vi "Level_DSP.vi"(8 "error in (no error)":errorcluster caption="에러 입력(에러 없음)", 9 "Curr":dbl, 10 "Volt":dbl, 11 "VISA resource name":refnum<visa-resource-name>) -> (0 "error out":errorcluster caption="에러 출력", 3 "VISA resource name Out":refnum<visa-resource-name>)   [LabVIEW 2019]
uses:
  f78cf197-b02f-4b1b-bb70-fad094e02e99.vi
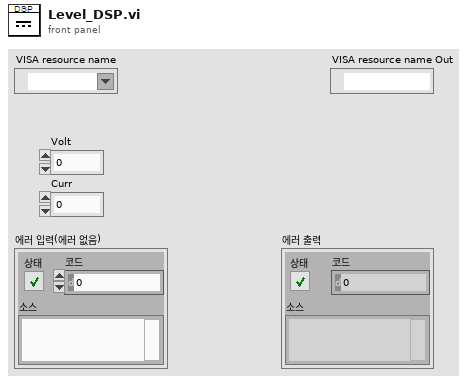
[diagram p1: front panel]
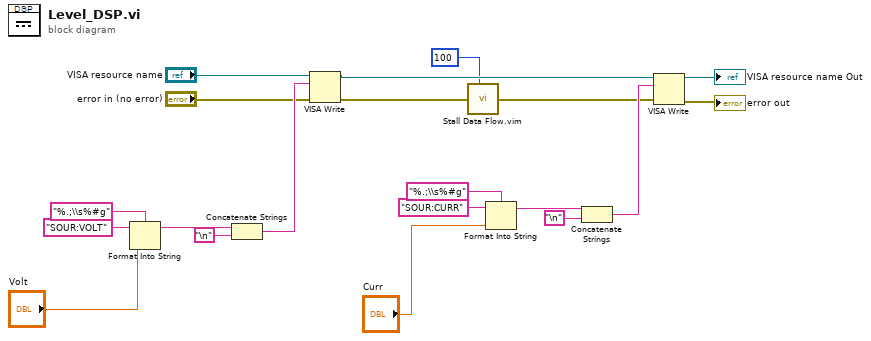
[diagram p0: block diagram]
diagram:
  n1 = Format Into String(format string="%.;\\s%#g", initial string="SOUR:VOLT", "Volt") -> (resulting string=w14:string)  [unwired: 1 in, 1 out]
  n2 = Concatenate Strings(w14, "\n") -> (w19:string)
  n3 = VISA Write(VISA resource name="VISA resource name", write buffer=w19, error in (no error)="error in (no error)") -> (VISA resource name out=w8:refnum<visa-resource-name>, error out=w7:errorcluster)  [unwired: 1 out]
  n4 = call "Stall Data Flow.vim"("value in"=w7, "milliseconds to wait"=u32 100) -> ("value out"=w2:errorcluster)  [unwired: 1 out]
  n5 = Format Into String(format string="%.;\\s%#g", initial string="SOUR:CURR", "Curr") -> (resulting string=w5:string)  [unwired: 1 in, 1 out]
  n6 = Concatenate Strings(w5, "\n") -> (w9:string)
  n7 = VISA Write(VISA resource name=w8, write buffer=w9, error in (no error)=w2) -> (VISA resource name out=→"VISA resource name Out":refnum<visa-resource-name>, error out=→"error out":errorcluster)  [unwired: 1 out]
